vi "lvstyx_write_path.vi"(7 "Log? (T)":bool=TRUE, 8 "error in (no error)":errorcluster, 9 "buf":string, 10 "path":string, 11 "client ptr":u32) -> (0 "error out":errorcluster, 1 "written len":i32, 3 "dup client ptr":u32)   [LabVIEW 2010, in "lib1299.lvlib"]
uses:
  lib1299.lvlib
  cstyx/win32/cstyx.dll
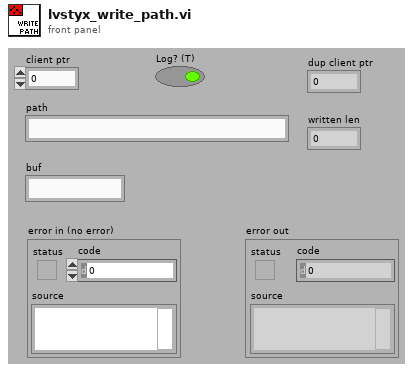
[diagram p1: front panel]
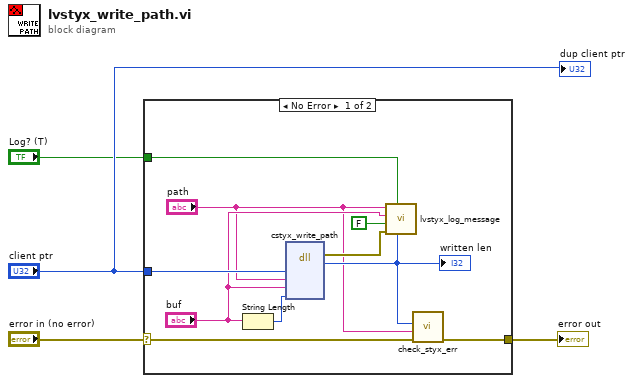
[diagram p0: block diagram]
diagram:
  n1 = case shown="No Error" "error in (no error)" {
    selector: "error in (no error)" -> [w10 w15]
    tunnel: "client ptr" -> [w12 _]
    tunnel: [w14 w15] -> w4
    tunnel: "Log? (T)" -> [w9 _]
    frame No Error {
      n2 = String Length(string="buf") -> (length=w13:i32)
      n3 = dll-call lib="C:/work/ads1299evm/lib_1299/Styx/cstyx/win32/cstyx.dll" fn="cstyx_write_path"("client"=w12, "path"="path", "buf"="buf", "len"=w13) -> (error out=w7:errorcluster, w6:i32)  [unwired: 7 in, 1 out]
      "written len" <- w6
      n4 = call "lvstyx_log_message.vi"("File Length"=w6, "Logging Enable (T)"=w9, "error in (no error)"=w7, "Read? (F)"=FALSE, "File value"="buf", "File Name"="path") -> ()  [unwired: 5 in, 1 out]
      n5 = call "check_styx_err.vi"("error in (no error)"=w10, "Additional Comment"="path", "return val"=w6) -> ("error out"=w14:errorcluster)  [unwired: 8 in]
    }
    frame Error {
    }
  }
  "error out" <- w4
  "dup client ptr" <- "client ptr"
